vi "incline.vi"(11 "Shared_strings":string[][](array[string])) -> ()   [LabVIEW 2018]
uses:
  Global Variables.vi
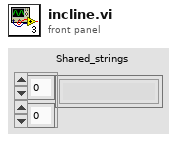
[diagram p1: front panel]
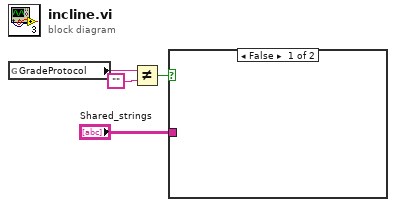
[diagram p0: block diagram]
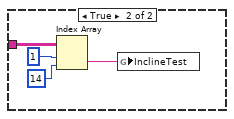
[diagram p2: hidden frame]
diagram:
  n1 = global read "Global Variables.vi" "GradeProtocol"() -> (w2:string)
  n2 = Not Equal?(x=w2, y="") -> (x != y?=w3:bool)
  n3 = case shown="False" w3 {
    tunnel: "Shared_strings" -> [_ w8]
    frame False {
    }
    frame True {
      n4 = Index Array(array=w8, index (row)=1, index (col)=14) -> (element=w5:string)
      n5 = global write "Global Variables.vi" "InclineTest"(w5) -> ()
    }
  }
